vi "Main.vi"() -> ()   [LabVIEW 2020]
uses:
  controls/message cluster.ctl
  <vilib>/Platform/TimedLoop/XDataNode/timing_clust.ctl
  <vilib>/Platform/TimedLoop/XDataNode/nitl_modes.ctl
  <vilib>/Platform/TimedLoop/XDataNode/wakeup.ctl
  <instrlib>/Marlin Instrument Driver/Public/controls/move parameters.ctl
  <instrlib>/Marlin Instrument Driver/Public/controls/axes.ctl
  <instrlib>/Marlin Instrument Driver/Public/controls/heater.ctl
  <vilib>/Utility/config.llb/Read Key (String).vi
  <vilib>/Utility/config.llb/Read Key (Double).vi
  <vilib>/Utility/config.llb/Write Key (String).vi
  <vilib>/Utility/config.llb/Write Key (Double).vi
  <vilib>/platform/TimedLoop/XDataNode/XDataNode.xnode
  <instrlib>/Marlin Instrument Driver/Marlin Instrument Driver.lvlib
  <vilib>/Utility/config.llb/NI_LVConfig.lvlib
  <vilib>/Platform/TimedLoop/XDataNode/XDNodeRunTimeDep.lvlib
panel:
  in  "Tab Control":T1(tab)
  in  "Disable steppers":bool
  in  "Chamber temp":enum16{"0", "40", "50", "60", "70", "80"}(ring) caption="Enum"
  in  "Bed temp":enum16{"0", "50", "60", "80", "100", "120"}(ring) caption="Enum"
  in  "Nozzle temp":T2(ring) caption="Enum"
  in  "Speed":u32=1000 caption="mm/min"
  in  "Distance":enum16{"0.1", "1", "10", "100"}(ring)=enum."10" caption="mm"
  in  "Fan control":u8(slide) caption="%" scale=0.0..255.0
  in  "Extrude":bool
  in  "Retract":bool
  in  "Home all":bool caption="ALL"
  in  "Home Z":bool
  in  "Z-":bool
  in  "Z+":bool
  in  "Home XY":bool
  in  "XY-":bool
  in  "X-":bool
  in  "XY+":bool
  in  "X-Y+":bool
  in  "Y-":bool
  in  "X+Y-":bool
  in  "X+":bool
  in  "Y+":bool
  in  "Monitor data":bool caption="Monitoring slows down communication"
  in  "Update frequency":u32=1000 caption="ms"
  out "Temperature Chart":dbl[][](graph)
  out "Z min":bool
  out "Y min":bool
  out "X min":bool
  out "Gcode array":string[](array[string])
  in  "Stop Gcode":bool
  in  "Pause Gcode":bool
  in  "Test mode":bool
  out "XY Graph":cluster{"X":dbl, "Y":dbl}[](graph)
  in  "Start Gcode":bool
  in  "Gcode file":path caption="Path"
  out "Position sent":dbl caption="Numeric"
  in  "Test mode":bool
  in  "Start torture":bool
  in  "Axle":enum16{"X", "Y", "Z"}(ring) caption="Enum"
  in  "Speed":u32(slide)=3000 caption="%" scale=0.0..9000.0
  in  "Distance":dbl(slide)=100.0 caption="%" scale=0.0..235.0
  out "Initialized":bool
  in  "Initialize":bool
  in  "Delete":bool
  in  "Save":bool
  in  "Z":dbl caption="Numeric"
  in  "Y":dbl caption="Numeric"
  in  "X":dbl caption="Build volume"
  in  "COM port":refnum<visa-resource-name>
  in  "3D printer":string(combo) caption="Combo Box"
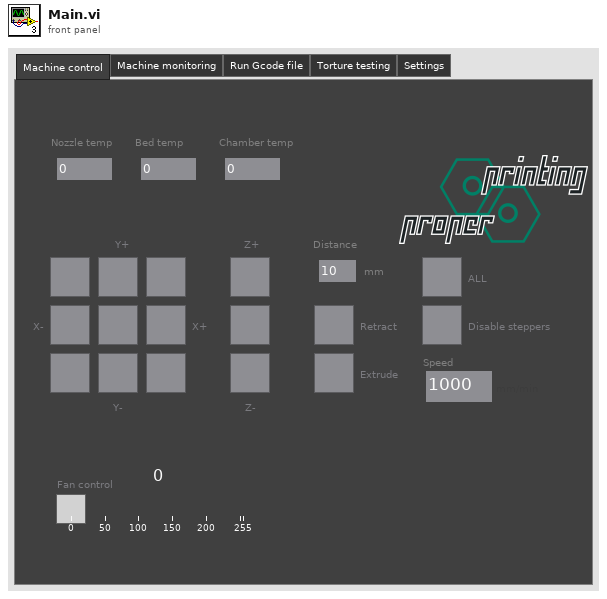
[diagram p1: front panel]
types:
  T1 = enum32{"Machine control", "Machine monitoring", "Run Gcode file", "Torture testing", "Settings"}
  T2 = enum16{"0", "100", "200", "230", "240", "260", "280", "290"}
  T3 = enum8{"Enabled", "Disabled", "Disabled and Grayed Out"}
  T4 = typedef "message cluster.ctl" = cluster{"message":string, "data":variant}
  T5 = typedef "XDNodeRunTimeDep.lvlib/timing_clust.ctl" = cluster{"Expected End [f-1]":u64, "Actual End [f-1]":u64, "Finished Late? [f-1]":bool, "Expected End [i-1]":u64, "Actual End [i-1]":u64, "Finished Late? [i-1]":bool, "Expected Start [i]":u64, "Actual Start [i]":u64, "Expected Start [f]":u64, "Actual Start [f]":u64, "Source Name":string, "Structure Name":string, "Period":i64, "Deadline":i64, "Offset":i64, "Start":i64, "Priority":i32, "Timeout":i32, "Mode":T6, "Wakeup Reason":T7, "Error":errorcluster, "Source Type":string, "Secondary Source Type":string, "Global End Time":u64, "Global Start Time":u64, "Frame Duration":u64, "Iteration Duration":u64, "Assigned CPU":i32, "I/O Scan Engine Mode":u32}
  T6 = typedef "XDNodeRunTimeDep.lvlib/nitl_modes.ctl" = enum32{"No Change", "Process missed periods, maintain original phase", "Discard missed periods, maintain original phase", "Process missed periods, ignore original phase", "Discard missed periods, ignore original phase"}
  T7 = typedef "XDNodeRunTimeDep.lvlib/wakeup.ctl" = enum32{"Normal", "Aborted", "Asynchronous wakeup", "Timing source error", "Timed loop error", "Timeout"}
  T8 = typedef "NI_LVConfig.lvlib/Config Data RefNum.ctl" = refnum<k1>
  T9 = typedef "Marlin Instrument Driver.lvlib/heater.ctl" = enum16{"Hot end", "Bed", "Chamber"}
  T10 = typedef "Marlin Instrument Driver.lvlib/move parameters.ctl" = cluster{"E":dbl, "F":dbl, "X":dbl, "Y":dbl, "Z":dbl}
  T11 = typedef "Marlin Instrument Driver.lvlib/axes.ctl" = cluster{"X":bool, "Y":bool, "Z":bool}
  T12 = typedef "Marlin Instrument Driver.lvlib/end stop status.ctl" = cluster{"x_min":bool, "y_min":bool, "z_min":bool}
  T13 = typedef "Marlin Instrument Driver.lvlib/temperatures.ctl" = cluster{"T":dbl, "T setpoint":dbl, "B":dbl, "B setpoint":dbl}
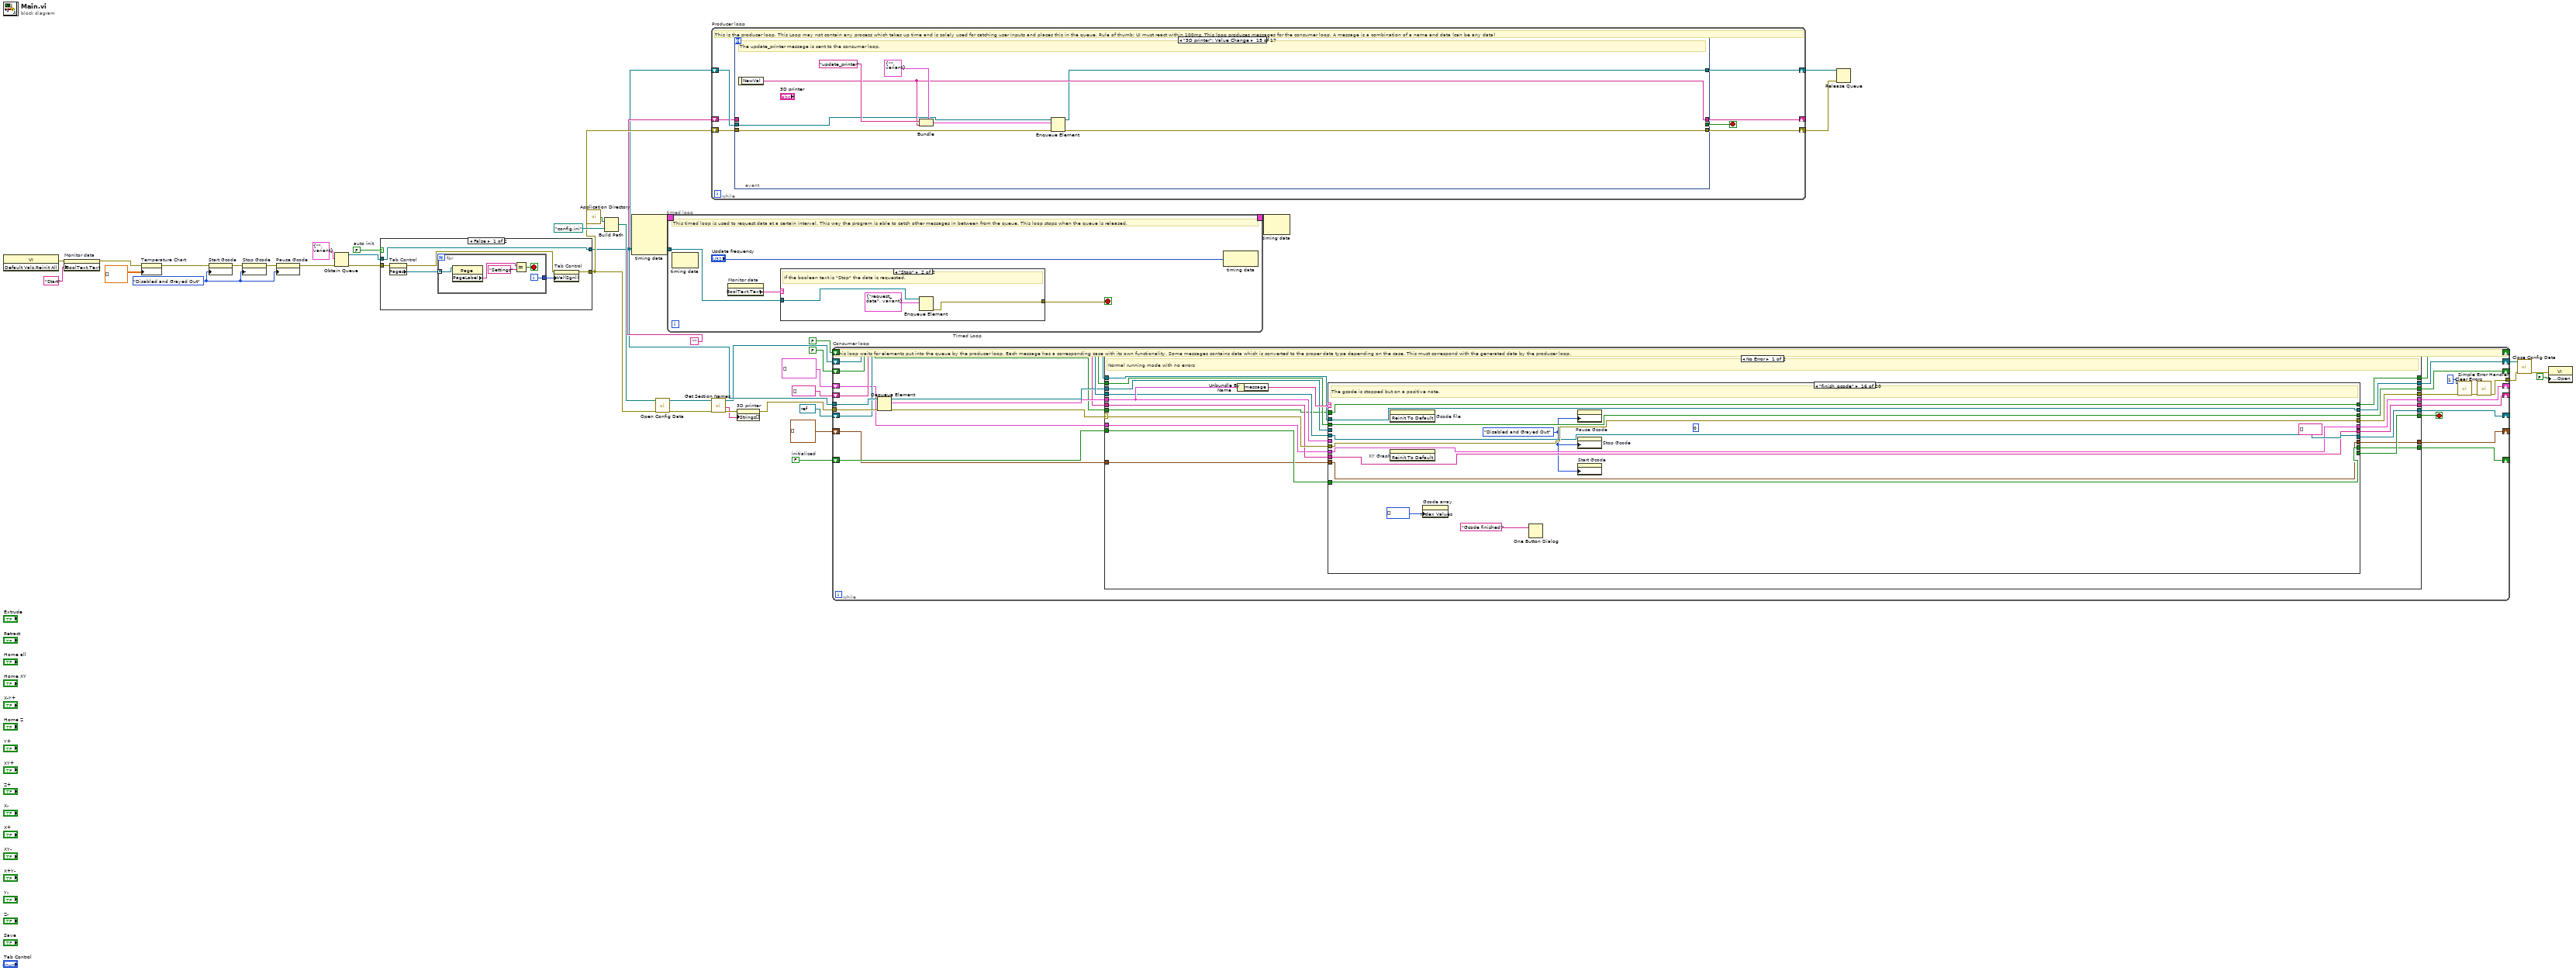
[diagram p0: block diagram]
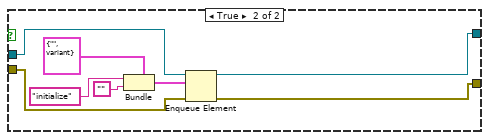
[diagram p2: hidden frame]
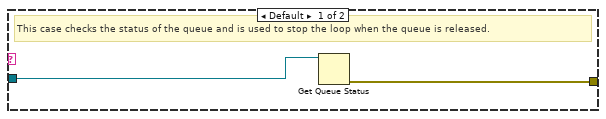
[diagram p3: hidden frame]
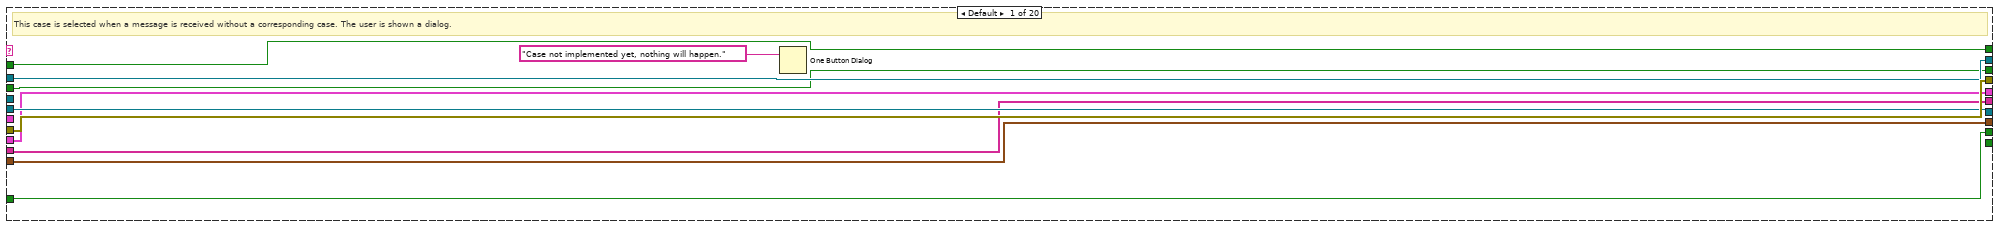
[diagram p4: hidden frame]
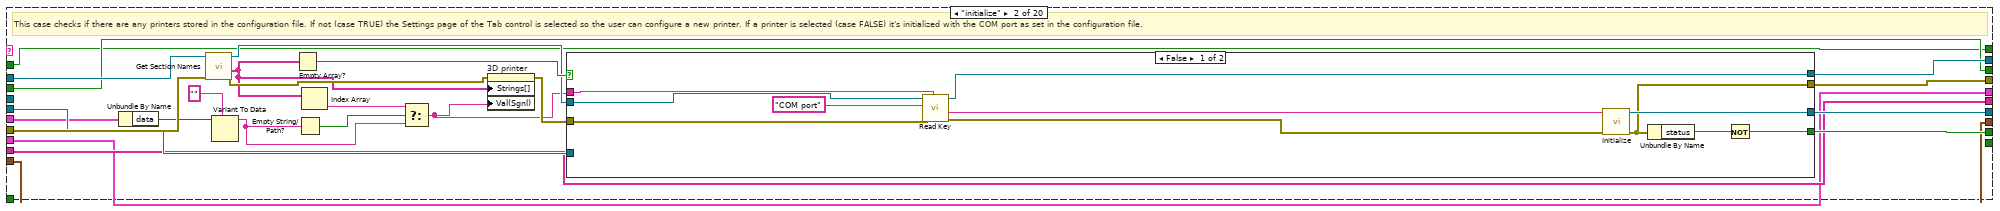
[diagram p5: hidden frame]
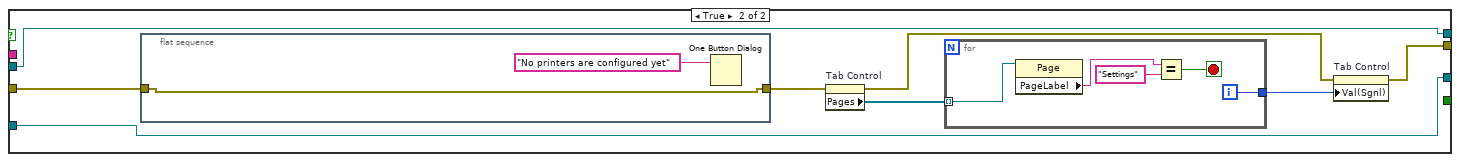
[diagram p6: hidden frame]
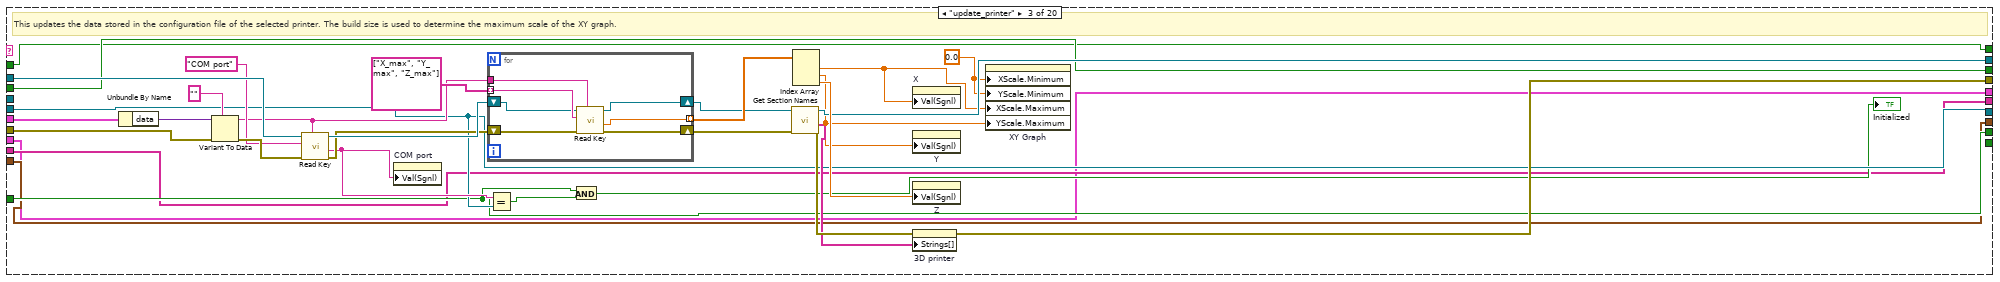
[diagram p7: hidden frame]
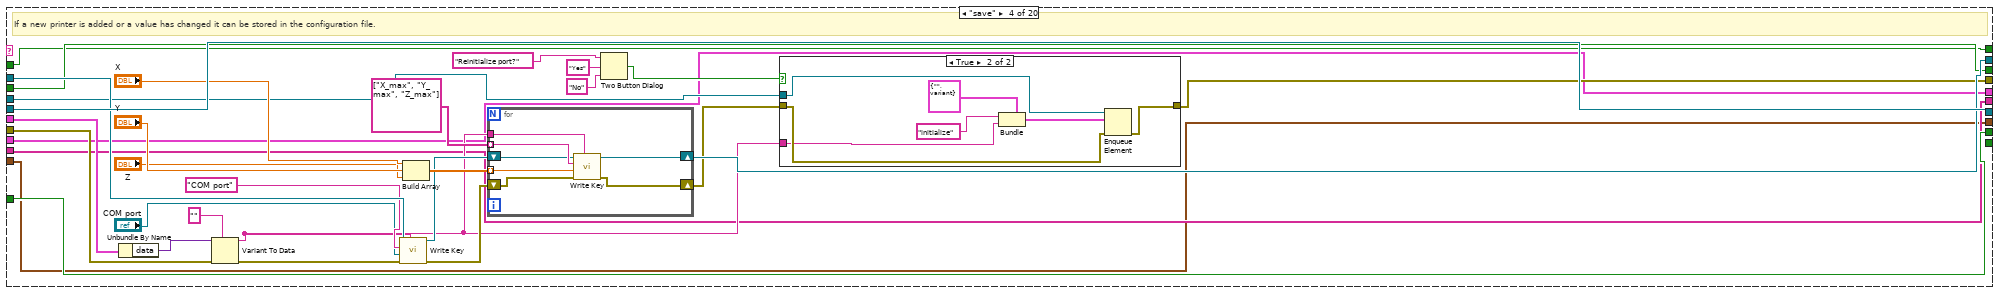
[diagram p8: hidden frame]
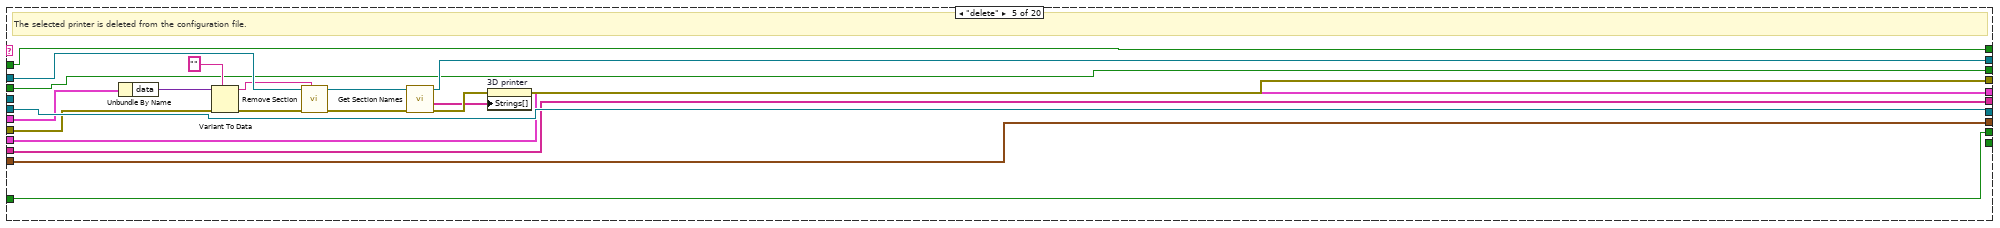
[diagram p10: hidden frame]
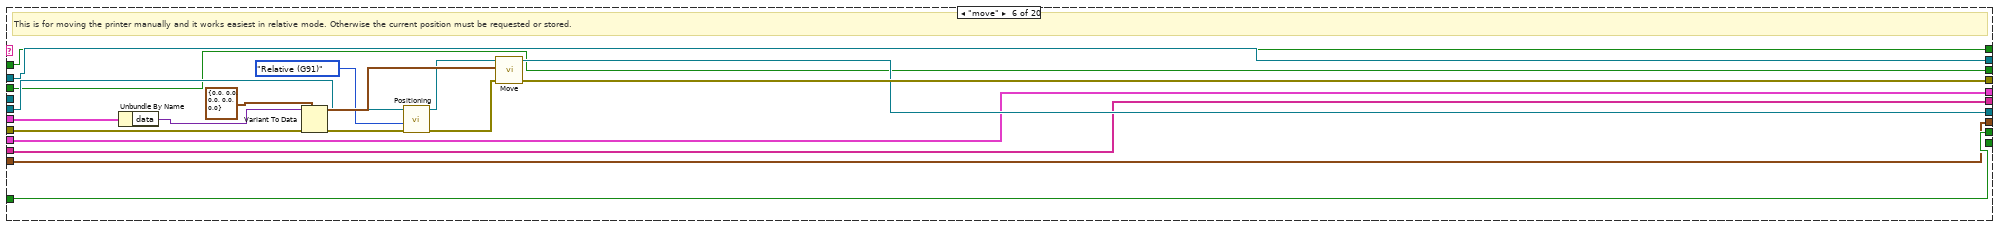
[diagram p11: hidden frame]
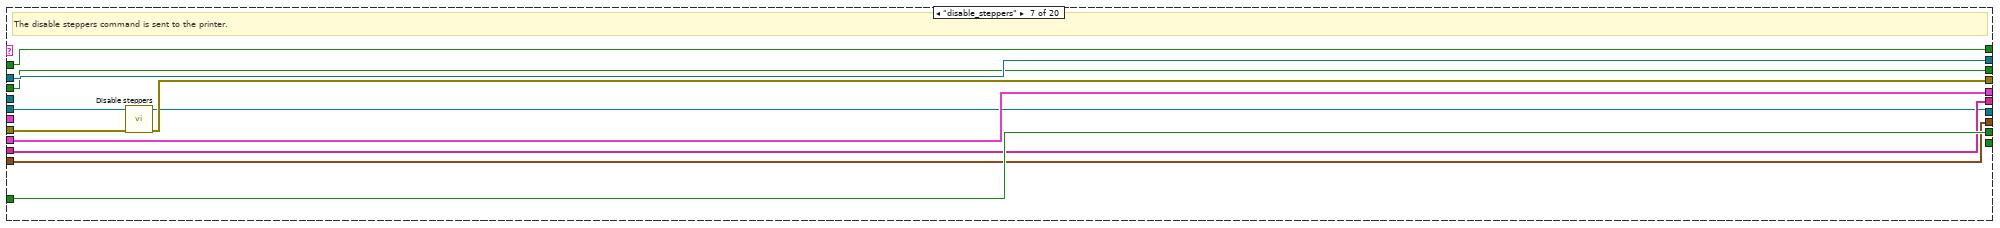
[diagram p12: hidden frame]
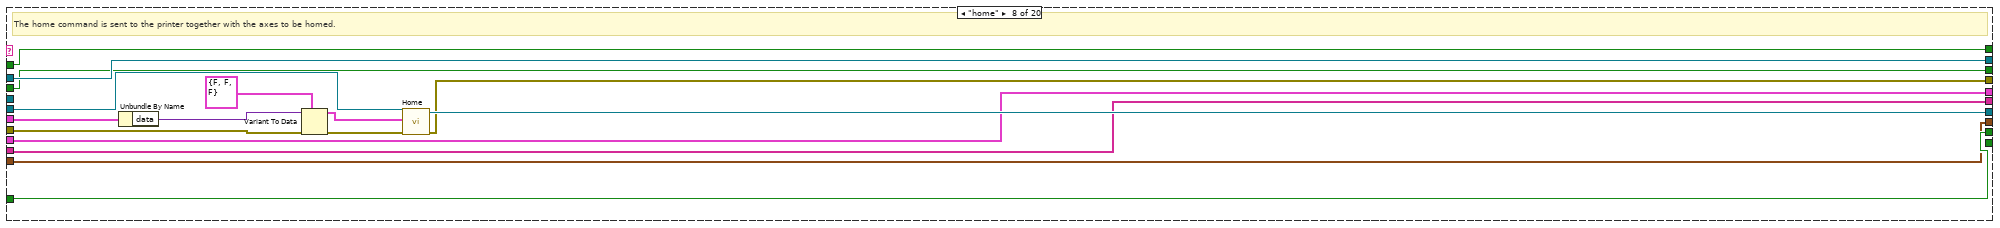
[diagram p13: hidden frame]
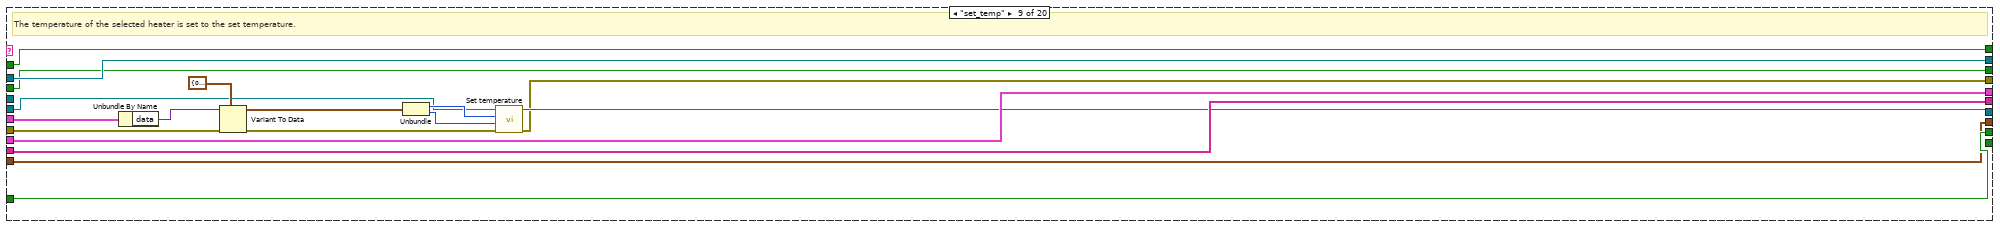
[diagram p14: hidden frame]
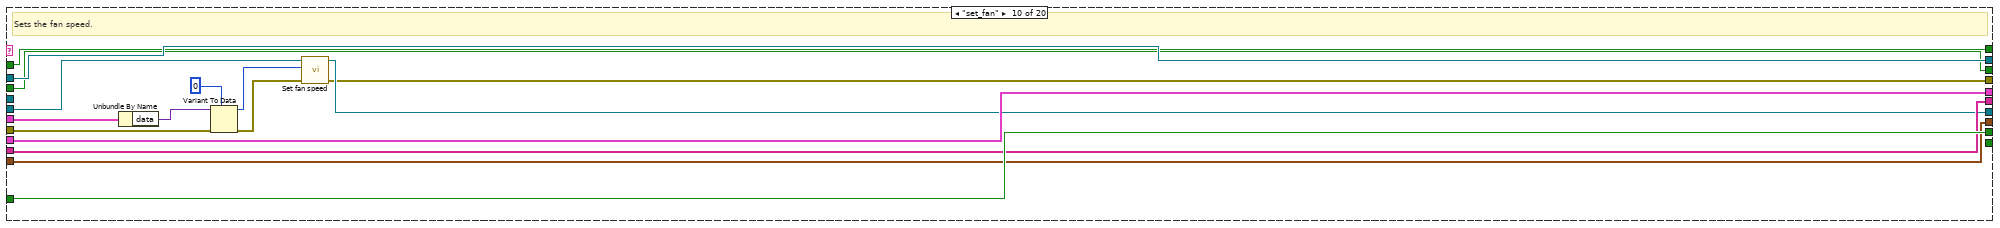
[diagram p15: hidden frame]
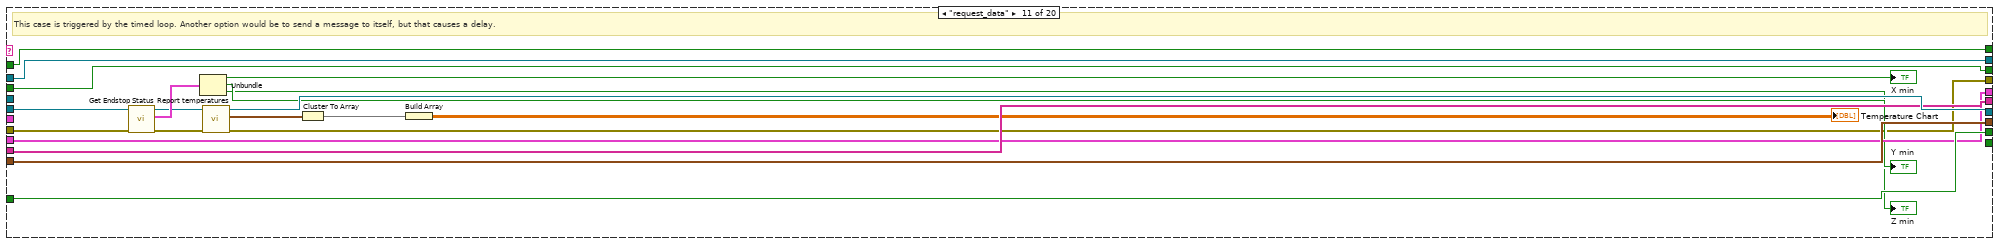
[diagram p16: hidden frame]
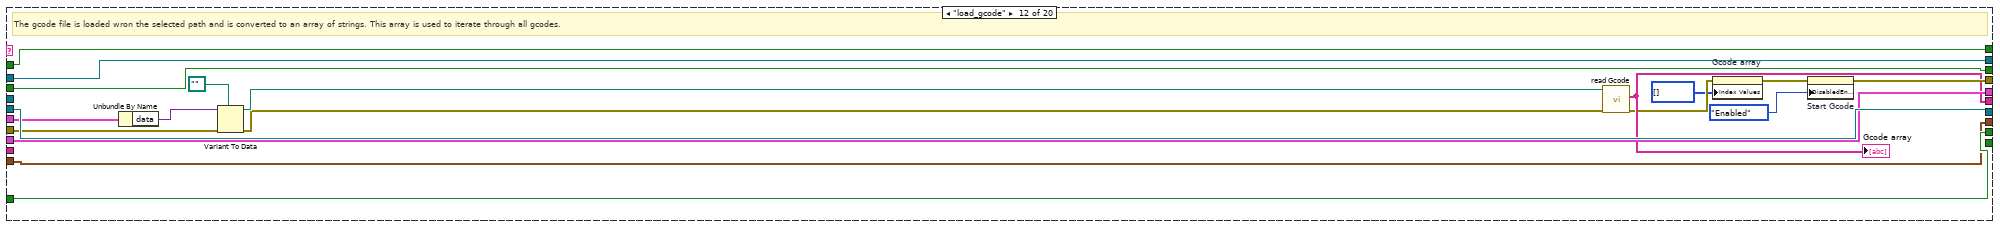
[diagram p17: hidden frame]
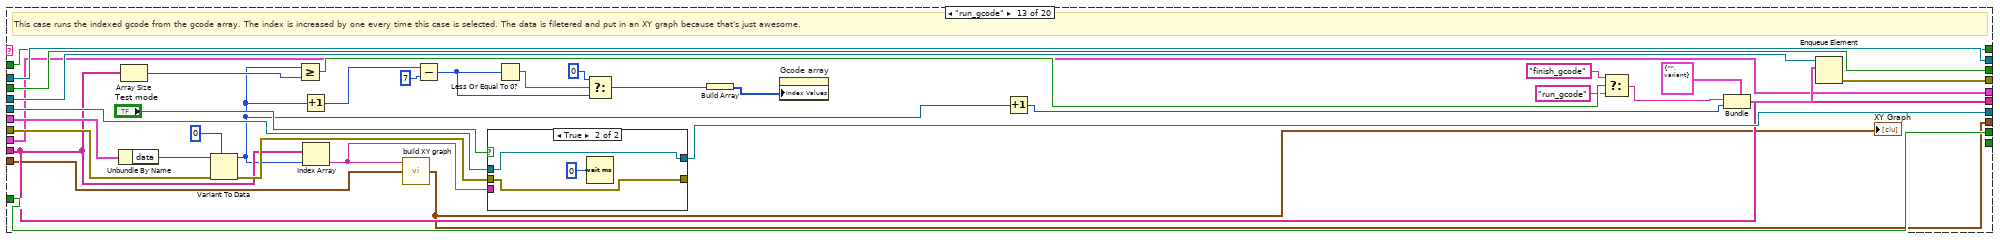
[diagram p18: hidden frame]
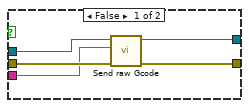
[diagram p19: hidden frame]
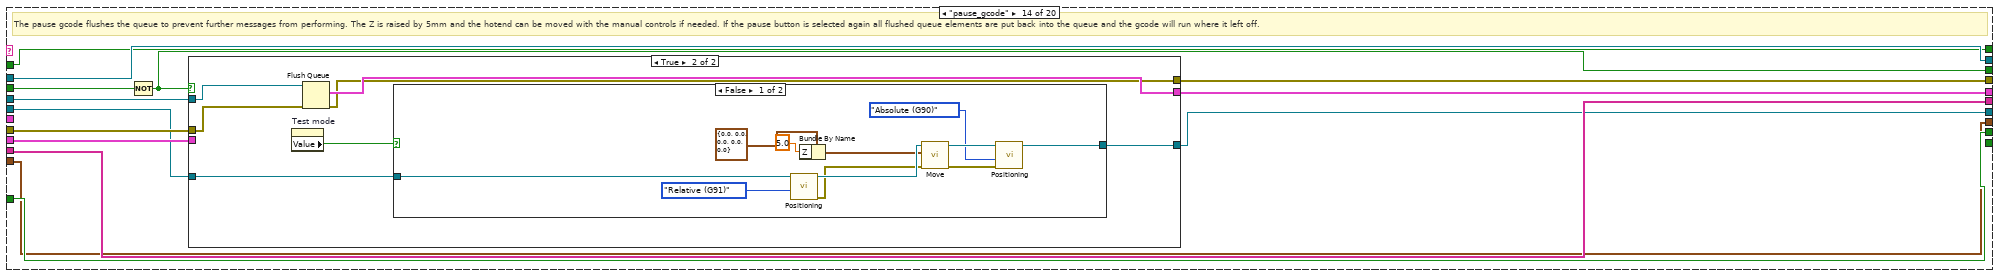
[diagram p20: hidden frame]
diagram:
  w15 = FALSE  # auto init
  w19 = T3."Disabled and Grayed Out" ("Disabled")
  w34 = FALSE  # initialized
  n1 = invoke class="VI" method="Default Vals.Reinit All"() -> (error out=w1:errorcluster)  [unwired: 3 in, 2 out]
  n2 = property on="Monitor data" class="Bool"(error in=w1, "BoolText.Text"="Start" ("Boolean Text.Text")) -> (error out=w11:errorcluster)  [unwired: 1 in, 1 out]
  n3 = property on="Temperature Chart" class="WFChart (strict)"(error in=w11, "History Data"=dbl[][] []) -> (error out=w14:errorcluster)  [unwired: 1 in, 1 out]
  n4 = property on="Start Gcode" class="Bool"(error in=w14, "DisabledEnum"=w19) -> (error out=w18:errorcluster)  [unwired: 1 in, 1 out]
  n5 = property on="Stop Gcode" class="Bool"(error in=w18, "DisabledEnum"=w19) -> (error out=w17:errorcluster)  [unwired: 1 in, 1 out]
  n6 = property on="Pause Gcode" class="Bool"(error in=w17, "DisabledEnum"=w19) -> (error out=w2:errorcluster)  [unwired: 1 in, 1 out]
  n7 = Obtain Queue(element data type=T4 {"message"="", "data"=variant}, error in (no error)=w2) -> (queue out=w37:refnum<queue>, error out=w36:errorcluster)  [unwired: 3 in, 1 out]
  n8 = case shown="False" w15 {
    tunnel: w37 -> [w46 w59]
    tunnel: w36 -> [w42 w58]
    tunnel: [w41 w57] -> w30
    tunnel: [w46 w52] -> w20
    frame False {
      n9 = property on="Tab Control" class="TabCtl (strict)"(error in=w42) -> (error out=w43:errorcluster, "Pages"=w44:refnum<vi>[])  [unwired: 1 in, 1 out]
      n10 = for {
        tunnel: w44 -> [w51] mode=indexing
        tunnel: [w47] -> w45
        i -> [w47]
        stop <- w48 stop-if-true
        n11 = property class="Page"(reference=w51) -> ("PageLabel"=w50:string)  [unwired: 1 in, 2 out]
        n12 = Equal?(x=w50, y="Settings") -> (x = y?=w48:bool)
      }
      n13 = property on="Tab Control" class="TabCtl (strict)"(error in=w43, "Val(Sgnl)"=w45) -> (error out=w41:errorcluster)  [unwired: 1 in, 1 out]
    }
    frame True {
      n14 = Bundle(cluster=T4 {"message"="", "data"=variant}, "message"="initialize", "data"="") -> (w53:T4)
      n15 = Enqueue Element(queue=w59, element=w53, error in (no error)=w58) -> (queue out=w52:refnum<queue>, error out=w57:errorcluster)  [unwired: 1 in, 1 out]
    }
  }
  n16 = call <vilib>:"Application Directory.vi"() -> ("Application Directory"=w33:path)
  n17 = Build Path(base path=w33, name or relative path=path "config.ini") -> (appended path=w31:path)
  n18 = node-c288() -> (w22:T5)  [unwired: 4 in]
  n19 = call <vilib>:"Open Config Data.vi"("error in (no error)"=w30, "configuration file path"=w31) -> ("error out"=w8:errorcluster, "refnum"=w7:T8)  [unwired: 7 in, 1 out]
  n20 = timed-loop "Timed Loop" {
    timing: w22 -> [_]
    timing-out: [_] -> w21
    tunnel: w20 -> [w62]
    stop <- w60 stop-if-true
    # "This timed loop is used to request data at a certain interval. This way the program is able to catch other messages in between from the queue. This loop stops when the queue is released."
    n21 = node-c288() -> ()  [unwired: 1 in, 1 out]
    n22 = property on="Monitor data" class="Bool"() -> ("BoolText.Text"=w61:string)  [unwired: 2 in, 2 out]
    n23 = case shown="\"Stop\"" w61 {
      tunnel: w62 -> [w64 w68]
      tunnel: [w65 w67] -> w60
      frame Default {
        # "This case checks the status of the queue and is used to stop the loop when the queue is released."
        n24 = Get Queue Status(queue=w64) -> (error out=w65:errorcluster)  [unwired: 2 in, 7 out]
      }
      frame "Stop" {
        # "If the boolean text is \"Stop\" the data is requested."
        n25 = Enqueue Element(queue=w68, element=T4 {"message"="request_data", "data"=variant}) -> (error out=w67:errorcluster)  [unwired: 2 in, 2 out]
      }
    }
    n26 = node-c288("Update frequency") -> ()  [unwired: 1 out]
  }
  n27 = while "Producer loop" {
    shift-right: [w76] -> w39
    shift-left: w30 -> [w77]
    shift-right: [w75] -> w38
    shift-left: w20 -> [w78]
    shift-right: [w74] -> _
    shift-left: "" -> [w73]
    stop <- w79 stop-if-true
    # "This is the producer loop. This Loop may not contain any process which takes up time and is solely used for catching user inputs and places this in the queue. Rule of thumb: UI must react within 100ms. This loop produces messages for the consumer loop. A message is a combination of a name and data (can be any data)"
    n28 = event shown="[14] \"3D printer\": Value Change" {
      selector: _ -> [_ _ _ _ _ _ _ _ _ _ _ _ _ _ _ _ _]
      dyn-events: _ -> [_ _ _ _ _ _ _ _ _ _ _ _ _ _ _ _ _]
      timeout: _ -> [_ _ _ _ _ _ _ _ _ _ _ _ _ _ _ _ _]
      tunnel: [_ _ _ _ _ _ _ _ _ _ _ _ _ _ _ _ TRUE] -> w79
      tunnel: w78 -> [w81 w87 w97 w125 w177 w187 w205 w219 w233 w242 w251 w270 w280 w296 w300 w308 w319]
      tunnel: w77 -> [w82 w86 w95 w120 w175 w185 w202 w217 w229 w239 w252 w268 w278 w294 w299 w307 w317]
      tunnel: [w82 w85 w94 w119 w174 w184 w201 w215 w224 w238 w246 w267 w277 w293 w298 w306 w316] -> w76
      tunnel: [w81 w84 w96 w121 w176 w186 w204 w218 w233 w240 w250 w269 w279 w295 w297 w305 w315] -> w75
      tunnel: [w80 w83 w107 w115 w179 w188 w211 w223 w235 w245 w254 w272 w281 w290 w301 w309 w314] -> w74
      tunnel: w73 -> [w80 w83 w107 w115 w179 w188 w211 w223 w235 w245 w254 w272 w281 w290 _ w309 w314]
      event Timeout {
        # "This event will never trigger (timeout = -1)"
        n29 = event-data() -> ()  [unwired: 1 in, 3 out]
      }
      event "Initialize": Value Change {
        # "The initialize message is sent to the consumer loop."
        n30 = event-data() -> ()  [unwired: 1 in, 6 out]
        n31 = Bundle(cluster=T4 {"message"="", "data"=variant}, "message"="initialize", "data"=w83) -> (w88:T4)
        n32 = Enqueue Element(queue=w87, element=w88, error in (no error)=w86) -> (queue out=w84:refnum<queue>, error out=w85:errorcluster)  [unwired: 1 in, 1 out]
      }
      event "Nozzle temp", "Bed temp", "Chamber temp": Value Change {
        # "This event looks at the lable of which input has changed which corresponds with a case. The data is sent together with the set_temp message to the consumer loop."
        n33 = event-data() -> ("CtlRef"=w106:refnum<vi>)  [unwired: 1 in]
        n34 = property class="Enum"(reference=w106) -> ("Label.Text"=w105:string, "Strings []"=w104:string[])  [unwired: 1 in, 2 out]
        n35 = case shown="\"Chamber temp\"" w105 {
          tunnel: ["Bed temp" "Chamber temp" "Nozzle temp"] -> w103
          tunnel: [heater."Bed" ("Heater") heater."Chamber" ("Heater") heater."Hot end" ("Heater")] -> w91
          frame "Bed temp" {
          }
          frame "Chamber temp" {
          }
          frame "Nozzle temp", Default {
          }
        }
        n36 = Index Array(array=w104, index=w103) -> (element=w102:string)
        n37 = Decimal String To Number(string=w102) -> (number=w101:i32)  [unwired: 2 in, 1 out]
        n38 = Bundle(cluster=cluster{"setpoint":i32, "Heater":T9} {"setpoint"=0, "Heater"=enum."Hot end"} ("output cluster"), "setpoint"=w101, "Heater"=w91) -> (w93:cluster{"setpoint":i32, "Heater":T9})
        n39 = Bundle(cluster=T4 {"message"="", "data"=variant}, "message"="set_temp", "data"=w93) -> (w98:T4)
        n40 = Enqueue Element(queue=w97, element=w98, error in (no error)=w95) -> (queue out=w96:refnum<queue>, error out=w94:errorcluster)  [unwired: 1 in, 1 out]
      }
      event "Y+", "X+", "X+Y-", "Y-", "X-Y+", "XY+", "X-", "XY-", "Z+", "Z-", "Extrude", "Retract": Value Change {
        # "Depending on which button is pressed the matching case is selected. This sends the value with the move message. This only works with relative positioning because the unused values are 0."
        n41 = event-data() -> ("CtlRef"=w130:refnum<vi>)  [unwired: 1 in]
        n42 = property class="Bool"(reference=w130) -> ("Label.Text"=w129:string)  [unwired: 1 in, 2 out]
        n43 = property on="Distance" class="Enum (strict)"() -> ("Strings []"=w128:string[])  [unwired: 2 in, 2 out]
        n44 = Index Array(array=w128, index="Distance") -> (element=w127:string)
        n45 = Fract/Exp String To Number(string=w127) -> (number=w126:dbl)  [unwired: 3 in, 1 out]
        n46 = case shown="\"X+Y-\"" w129 {
          tunnel: w126 -> [_ w132 w135 w138 w141 w145 w149 w152 w156 w159 w163 w167 w171]
          tunnel: [_ w131 w134 w137 w142 w146 w150 w153 w157 w161 w165 w168 w172] -> w118
          frame Default {
          }
          frame "X+" {
            n47 = Bundle By Name(cluster=T10 {"E"=0.0, "F"=0.0, "X"=0.0, "Y"=0.0, "Z"=0.0} ("Distances"), "X"=w132) -> (w131:T10)
          }
          frame "Y+" {
            n48 = Bundle By Name(cluster=T10 {"E"=0.0, "F"=0.0, "X"=0.0, "Y"=0.0, "Z"=0.0} ("Distances"), "Y"=w135) -> (w134:T10)
          }
          frame "Z+" {
            n49 = Bundle By Name(cluster=T10 {"E"=0.0, "F"=0.0, "X"=0.0, "Y"=0.0, "Z"=0.0} ("Distances"), "Z"=w138) -> (w137:T10)
          }
          frame "X-" {
            n50 = Negate(x=w141) -> (-x=w140:dbl)
            n51 = Bundle By Name(cluster=T10 {"E"=0.0, "F"=0.0, "X"=0.0, "Y"=0.0, "Z"=0.0} ("Distances"), "X"=w140) -> (w142:T10)
          }
          frame "Y-" {
            n52 = Negate(x=w145) -> (-x=w144:dbl)
            n53 = Bundle By Name(cluster=T10 {"E"=0.0, "F"=0.0, "X"=0.0, "Y"=0.0, "Z"=0.0} ("Distances"), "Y"=w144) -> (w146:T10)
          }
          frame "Z-" {
            n54 = Negate(x=w149) -> (-x=w148:dbl)
            n55 = Bundle By Name(cluster=T10 {"E"=0.0, "F"=0.0, "X"=0.0, "Y"=0.0, "Z"=0.0} ("Distances"), "Z"=w148) -> (w150:T10)
          }
          frame "XY+" {
            n56 = Bundle By Name(cluster=T10 {"E"=0.0, "F"=0.0, "X"=0.0, "Y"=0.0, "Z"=0.0} ("Distances"), "X"=w152, "Y"=w152) -> (w153:T10)
          }
          frame "XY-" {
            n57 = Negate(x=w156) -> (-x=w155:dbl)
            n58 = Bundle By Name(cluster=T10 {"E"=0.0, "F"=0.0, "X"=0.0, "Y"=0.0, "Z"=0.0} ("Distances"), "X"=w155, "Y"=w155) -> (w157:T10)
          }
          frame "X+Y-" {
            n59 = Negate(x=w159) -> (-x=w160:dbl)
            n60 = Bundle By Name(cluster=T10 {"E"=0.0, "F"=0.0, "X"=0.0, "Y"=0.0, "Z"=0.0} ("Distances"), "X"=w159, "Y"=w160) -> (w161:T10)
          }
          frame "X-Y+" {
            n61 = Negate(x=w163) -> (-x=w164:dbl)
            n62 = Bundle By Name(cluster=T10 {"E"=0.0, "F"=0.0, "X"=0.0, "Y"=0.0, "Z"=0.0} ("Distances"), "X"=w164, "Y"=w163) -> (w165:T10)
          }
          frame "Extrude" {
            n63 = Bundle By Name(cluster=T10 {"E"=0.0, "F"=0.0, "X"=0.0, "Y"=0.0, "Z"=0.0} ("Distances"), "E"=w167) -> (w168:T10)
          }
          frame "Retract" {
            n64 = Negate(x=w171) -> (-x=w170:dbl)
            n65 = Bundle By Name(cluster=T10 {"E"=0.0, "F"=0.0, "X"=0.0, "Y"=0.0, "Z"=0.0} ("Distances"), "E"=w170) -> (w172:T10)
          }
        }
        n66 = Bundle By Name(cluster=w118, "F"="Speed") -> (w117:T10)
        n67 = Bundle(cluster=T4 {"message"="", "data"=variant}, "message"="move", "data"=w117) -> (w124:T4)
        n68 = Enqueue Element(queue=w125, element=w124, error in (no error)=w120) -> (queue out=w121:refnum<queue>, error out=w119:errorcluster)  [unwired: 1 in, 1 out]
      }
      event "Disable steppers": Value Change {
        # "The disable_steppers message is sent to the consumer loop."
        n69 = event-data() -> ()  [unwired: 1 in, 6 out]
        n70 = Enqueue Element(queue=w177, element=T4 {"message"="disable_steppers", "data"=variant}, error in (no error)=w175) -> (queue out=w176:refnum<queue>, error out=w174:errorcluster)  [unwired: 1 in, 1 out]
      }
      event "Start torture": Value Change {
        # "Depending on the boolean text the start_torture or stop_torture  message is sent to the consumer loop. The boolean text is changed from start to stop and vice versa when pressed."
        n71 = event-data() -> ("CtlRef"=w183:refnum<vi>)  [unwired: 1 in, 5 out]
        n72 = property class="Bool"(reference=w183) -> (reference out=w181:refnum<vi>, "BoolText.Text"=w182:string)  [unwired: 1 in, 1 out]
        n73 = case shown="\"Start\"" w182 {
          tunnel: w187 -> [w193 w199]
          tunnel: [w192 w198] -> w186
          tunnel: w185 -> [w191 w197]
          tunnel: [w190 w196] -> w184
          tunnel: ["Stop" "Start"] -> w180
          frame "Start" {
            n74 = Enqueue Element(queue=w193, element=T4 {"message"="start_torture", "data"=variant}, error in (no error)=w191) -> (queue out=w192:refnum<queue>, error out=w190:errorcluster)  [unwired: 1 in, 1 out]
          }
          frame "Stop", Default {
            n75 = Enqueue Element At Opposite End(queue=w199, element=T4 {"message"="stop_torture", "data"=variant}, error in (no error)=w197) -> (queue out=w198:refnum<queue>, error out=w196:errorcluster)  [unwired: 1 in, 1 out]
          }
        }
        n76 = property class="Bool"(reference=w181, "BoolText.Text"=w180) -> ()  [unwired: 1 in, 2 out]
      }
      event "Home XY", "Home Z", "Home all": Value Change {
        # "The home message is sent to the consumer loop together with the data which tells which axes to home."
        n77 = event-data() -> ("CtlRef"=w210:refnum<vi>)  [unwired: 1 in]
        n78 = property class="Bool"(reference=w210) -> ("Label.Text"=w209:string)  [unwired: 1 in, 2 out]
        n79 = case shown="\"Home Z\"" w209 {
          tunnel: [T11 {"X"=TRUE, "Y"=TRUE, "Z"=TRUE} ("Axes") T11 {"X"=TRUE, "Y"=TRUE, "Z"=FALSE} ("Axes") T11 {"X"=FALSE, "Y"=FALSE, "Z"=TRUE} ("Axes")] -> w203
          frame "Home all", Default {
          }
          frame "Home XY" {
          }
          frame "Home Z" {
          }
        }
        n80 = Bundle(cluster=T4 {"message"="", "data"=variant}, "message"="home", "data"=w203) -> (w206:T4)
        n81 = Enqueue Element(queue=w205, element=w206, error in (no error)=w202) -> (queue out=w204:refnum<queue>, error out=w201:errorcluster)  [unwired: 1 in, 1 out]
      }
      event "Fan control": Value Change {
        # "The set_fan message is sent to the consumer loop. The NewVal is used and the event is triggered immediately when the Fan control slider is moved. This slows down communication and should therefore not be performed when a Gcode is running."
        n82 = event-data() -> ("NewVal"=w216:u8)  [unwired: 1 in]
        n83 = Bundle(cluster=T4 {"message"="", "data"=variant}, "message"="set_fan", "data"=w216) -> (w220:T4)
        n84 = Enqueue Element(queue=w219, element=w220, error in (no error)=w217) -> (queue out=w218:refnum<queue>, error out=w215:errorcluster)  [unwired: 1 in, 1 out]
      }
      event "Monitor data": Value Change {
        w227 = "Start" ("y")
        # "This event changes the boolean text of the Monitor data button from Start to Stop and vice versa. This is used to enable or disable the timed loop data request."
        n85 = event-data() -> ("CtlRef"=w234:refnum<vi>)  [unwired: 1 in, 2 out]
        n86 = property class="Bool"(reference=w234, error in=w229) -> (reference out=w231:refnum<vi>, error out=w230:errorcluster, "BoolText.Text"=w232:string)
        n87 = Equal?(x=w232, y=w227) -> (x = y?=w228:bool)
        n88 = Select(t="Stop", s=w228, f=w227) -> (s? t:f=w225:string)
        n89 = property class="Bool"(reference=w231, error in=w230, "BoolText.Text"=w225) -> (error out=w224:errorcluster)  [unwired: 1 out]
      }
      event "Gcode file": Value Change {
        # "The load_gcode message is sent to the consumer loop together with the selected path."
        n90 = event-data() -> ("NewVal"=w237:path)  [unwired: 1 in]
        n91 = Strip Path(path=w237) -> (name=w236:string)  [unwired: 1 out]
        n92 = property on="Gcode file" class="Path"("Text.Text"=w236) -> ()  [unwired: 2 in, 2 out]
        n93 = Bundle(cluster=T4 {"message"="", "data"=variant} ("element"), "message"="load_gcode", "data"=w237) -> (w241:T4)
        n94 = Enqueue Element(queue=w242, element=w241, error in (no error)=w239) -> (queue out=w240:refnum<queue>, error out=w238:errorcluster)  [unwired: 1 in, 1 out]
      }
      event "Start Gcode": Value Change {
        # "The run_gcode message is sent to the consumer loop after the user confirms the message. The current index of the Gcode array (first array element is 0) is sent as data."
        n95 = event-data() -> ()  [unwired: 1 in, 4 out]
        n96 = Two Button Dialog(message="Run selected program?", 1:"No" ("F button name (\"Cancel\")"), 2:"Yes" ("T button name (\"OK\")")) -> (T button?=w249:bool)
        n97 = case shown="True" w249 {
          tunnel: w252 -> [w255 w263]
          tunnel: w251 -> [w256 w262]
          tunnel: [w256 w261] -> w250
          tunnel: [w255 w259] -> w246
          frame False {
          }
          frame True {
            w257 = T3."Enabled" ("Disabled")
            n98 = property on="Stop Gcode" class="Bool"("DisabledEnum"=w257) -> ()  [unwired: 2 in, 2 out]
            n99 = property on="Pause Gcode" class="Bool"("DisabledEnum"=w257) -> ()  [unwired: 2 in, 2 out]
            n100 = Bundle(cluster=T4 {"message"="", "data"=variant} ("element"), "message"="run_gcode", "data"=0) -> (w264:T4)
            n101 = property on="Start Gcode" class="Bool"("DisabledEnum"=T3."Disabled and Grayed Out" ("Disabled")) -> ()  [unwired: 2 in, 2 out]
            n102 = Enqueue Element(queue=w262, element=w264, error in (no error)=w263) -> (queue out=w261:refnum<queue>, error out=w259:errorcluster)  [unwired: 1 in, 1 out]
          }
        }
      }
      event "Pause Gcode": Value Change {
        # "The pause_gcode message is sent to the consumer loop."
        n103 = event-data() -> ()  [unwired: 1 in, 1 out]
        n104 = Enqueue Element(queue=w270, element=T4 {"message"="pause_gcode", "data"=variant}, error in (no error)=w268) -> (queue out=w269:refnum<queue>, error out=w267:errorcluster)  [unwired: 1 in, 1 out]
      }
      event "Stop Gcode": Value Change {
        # "The stop_gcode message is sent to the consumer loop after the user confirms the message."
        n105 = event-data() -> ()  [unwired: 1 in, 1 out]
        n106 = Two Button Dialog(message="Stop current running program?", 1:"No" ("F button name (\"Cancel\")"), 2:"Yes" ("T button name (\"OK\")")) -> (T button?=w273:bool)
        n107 = case shown="True" w273 {
          tunnel: w280 -> [w283 w287]
          tunnel: [w283 w286] -> w279
          tunnel: w278 -> [w282 w285]
          tunnel: [w282 w284] -> w277
          frame False {
          }
          frame True {
            n108 = Enqueue Element At Opposite End(queue=w287, element=T4 {"message"="stop_gcode", "data"=variant}, error in (no error)=w285) -> (queue out=w286:refnum<queue>, error out=w284:errorcluster)  [unwired: 1 in, 1 out]
          }
        }
      }
      event "Save": Value Change {
        # "The save message is sent to the consumer loop."
        n109 = event-data() -> ()  [unwired: 1 in, 6 out]
        n110 = Bundle(cluster=T4 {"message"="", "data"=variant}, "message"="save", "data"=w290) -> (w289:T4)
        n111 = Enqueue Element(queue=w296, element=w289, error in (no error)=w294) -> (queue out=w295:refnum<queue>, error out=w293:errorcluster)  [unwired: 1 in, 1 out]
      }
      event "3D printer": Value Change {
        # "The update_printer message is sent to the consumer loop."
        n112 = event-data() -> ("NewVal"=w301:string)  [unwired: 1 in]
        n113 = Bundle(cluster=T4 {"message"="", "data"=variant}, "message"="update_printer", "data"=w301) -> (w302:T4)
        n114 = Enqueue Element(queue=w300, element=w302, error in (no error)=w299) -> (queue out=w297:refnum<queue>, error out=w298:errorcluster)  [unwired: 1 in, 1 out]
      }
      event "Delete": Value Change {
        # "The delete message is sent to the consumer loop."
        n115 = event-data() -> ()  [unwired: 1 in, 1 out]
        n116 = Bundle(cluster=T4 {"message"="", "data"=variant}, "message"="delete", "data"=w309) -> (w310:T4)
        n117 = Enqueue Element(queue=w308, element=w310, error in (no error)=w307) -> (queue out=w305:refnum<queue>, error out=w306:errorcluster)  [unwired: 1 in, 1 out]
      }
      event Panel Close? {
        # "The close message is sent to the consumer loop when the front panel is closed by the user. The message is discarded so the program can close the port first. The program quits after all loops are stopped."
        n118 = event-data() -> ()  [unwired: 1 in, 4 out]
        n119 = Enqueue Element(queue=w319, element=T4 {"message"="close", "data"=variant}, error in (no error)=w317) -> (queue out=w315:refnum<queue>, error out=w316:errorcluster)  [unwired: 1 in, 1 out]
        n120 = event-data("Discard?"=TRUE) -> ()  [unwired: 1 in, 1 out]
      }
    }
  }
  n121 = call <vilib>:"Get Section Names.vi"("error in (no error)"=w8, "refnum"=w7) -> ("error out"=w4:errorcluster, "section names"=w3:string[], "refnum out"=w6:T8)  [unwired: 7 in]
  n122 = property on="3D printer" class="CmbBox"(error in=w4, "Strings[]"=w3) -> (error out=w5:errorcluster)  [unwired: 1 in, 1 out]
  n123 = while "Consumer loop" {
    tunnel: w20 -> [w346]
    shift-right: [w341] -> _
    shift-left: refnum<visa-resource-name> refnum ("VISA resource name out") -> [w339]
    shift-right: [w340] -> w29
    shift-left: w6 -> [w338]
    shift-right: [w337] -> _
    shift-left: w34 -> [w336]
    shift-right: [w334] -> _
    shift-left: string[] [] ("Gcode Array") -> [w333]
    shift-right: [w331] -> _
    shift-left: cluster{"X":dbl, "Y":dbl}[] [] ("XY Graph 2") -> [w332]
    shift-right: [w326] -> _
    shift-left: FALSE -> [w327]
    shift-right: [w325] -> _
    shift-left: T4[] [] ("remaining elements") -> [w324]
    tunnel: w5 -> [w342]
    tunnel: [w323] -> w27
    shift-right: [w321] -> _
    shift-left: FALSE -> [w322]
    stop <- w344 stop-if-true
    # "This loop waits for elements put into the queue by the producer loop. Each message has a corresponding case with its own functionality. Some messages contains data which is converted to the proper data type depending on the case. This must correspond with the generated data by the producer loop."
    n124 = Dequeue Element(queue=w346, error in (no error)=w342) -> (queue out=w335:refnum<queue>, element=w345:T4, error out=w343:errorcluster)  [unwired: 1 in, 1 out]
    n125 = case shown="No Error" w343 {
      selector: w343 -> [w365 _]
      tunnel: w345 -> [w367 _]
      tunnel: [w366 FALSE] -> w344
      tunnel: [w364 w899] -> w341
      tunnel: [w363 w898] -> w340
      tunnel: w339 -> [w362 w899]
      tunnel: w338 -> [w361 w898]
      tunnel: [w360 _] -> w337
      tunnel: w336 -> [w359 _]
      tunnel: w335 -> [w358 w890]
      tunnel: [w357 w889] -> w330
      tunnel: [w356 w896] -> w334
      tunnel: w333 -> [w355 w896]
      tunnel: w332 -> [w354 w895]
      tunnel: [w353 w895] -> w331
      tunnel: w327 -> [w352 w894]
      tunnel: [w351 w894] -> w326
      tunnel: [w350 w893] -> w325
      tunnel: w324 -> [w349 w893]
      tunnel: w322 -> [w348 w892]
      tunnel: [w347 w892] -> w321
      frame No Error {
        # "Normal running mode with no errors"
        n126 = Unbundle By Name(w367) -> ("message"=w368:string)
        n127 = case shown="\"finish_gcode\"" w368 {
          tunnel: w367 -> [_ w391 w458 w482 w525 w552 _ w574 w591 w607 _ w649 w684 _ _ _ _ _ _ _]
          tunnel: [_ _ _ _ _ _ _ _ _ _ _ _ _ _ _ _ _ _ _ TRUE] -> w366
          tunnel: [w378 w399 w442 w483 w519 w548 w555 w569 w583 w603 w614 w639 w676 w699 w742 w760 w764 w823 w867 w878] -> w357
          tunnel: w365 -> [w378 w396 w457 w479 w528 w547 w556 w575 w582 w602 w616 w644 w683 w700 w743 w760 w769 w828 w868 w879]
          tunnel: [w376 w400 w440 w498 w533 w546 w554 w570 w584 w604 w630 w652 w679 w696 w748 w759 w762 w826 w877 w880] -> w364
          tunnel: [w377 w398 w444 w486 w520 w545 w563 w579 w597 w613 w633 w651 w687 w709 w747 w758 w776 w836 w876 w887] -> w363
          tunnel: w362 -> [w376 w394 w440 w498 w533 w541 w557 w577 w585 w605 w631 w652 w681 w697 w748 w759 w770 w827 w877 w880]
          tunnel: w361 -> [w377 w395 w455 w496 w531 w545 w563 w579 w597 w613 w633 w651 w687 w709 w747 w758 w776 w836 w876 w887]
          tunnel: [w375 w397 w439 w497 w532 w544 w562 w578 w596 w612 w632 w650 w686 w708 w746 w757 w775 w835 w875 w886] -> w360
          tunnel: w359 -> [w375 _ w439 w497 w532 w544 w562 w578 w596 w612 w632 w650 w686 w708 w746 w757 w775 w835 w875 w886]
          tunnel: w358 -> [_ _ _ w485 _ _ _ _ _ _ _ _ w675 w704 w744 _ w766 w822 w869 _]
          tunnel: [w374 w383 w436 w472 w518 w538 w561 w568 w595 w611 w629 w637 w674 w707 _ w756 w774 w834 w874 w885] -> w356
          tunnel: w355 -> [w374 w383 w436 w472 w518 w538 w561 w568 w595 w611 w629 _ w674 w707 _ w756 w774 w834 w874 w885]
          tunnel: w354 -> [w373 w382 w435 w471 w517 w537 w560 w567 w594 w610 w628 w643 w667 w706 w745 w754 w773 w833 w873 w884]
          tunnel: [w373 w382 w435 w471 w517 w537 w560 w567 w594 w610 w628 w643 w665 w706 w745 w754 w773 w833 w873 w884] -> w353
          tunnel: w352 -> [w372 w381 w431 w470 w516 w536 w559 w566 w593 w609 w627 w642 w657 w705 w741 w753 w772 w832 w872 w883]
          tunnel: [w372 w381 w431 w470 w516 w536 w559 w566 w593 w609 w627 w642 w657 w703 w741 w753 w772 w832 w872 w883] -> w351
          tunnel: [w371 w380 w430 w469 w515 w535 w558 w565 w592 w608 w626 w641 w656 w702 _ w752 w771 w831 w871 w882] -> w350
          tunnel: w349 -> [w371 w380 w430 w469 w515 w535 w558 w565 w592 w608 w626 w641 w656 w701 _ w752 w771 w831 w871 w882]
          tunnel: w348 -> [w370 w379 w429 w468 w514 w534 w553 w564 w580 w598 w615 w638 w655 w698 w739 w750 _ w816 w870 w881]
          tunnel: [w370 w379 w429 w468 w514 w534 w553 w564 w580 w598 w615 w638 w655 w698 w739 w750 FALSE w815 w870 w881] -> w347
          frame Default {
            # "This case is selected when a message is received without a corresponding case. The user is shown a dialog."
            n128 = One Button Dialog(message="Case not implemented yet, nothing will happen.") -> ()  [unwired: 1 in, 1 out]
          }
          frame "initialize" {
            # "This case checks if there are any printers stored in the configuration file. If not (case TRUE) the Settings page of the Tab control is selected so the user can configure a new printer. If a printer is selected (case FALSE) it's initialized with the COM port as set in the configuration file."
            n129 = Unbundle By Name(w391) -> ("data"=w393:variant)
            n130 = call <vilib>:"Get Section Names.vi"("error in (no error)"=w396, "refnum"=w395) -> ("error out"=w388:errorcluster, "section names"=w386:string[], "refnum out"=w401:T8)  [unwired: 7 in]
            n131 = Variant To Data(type="", Variant=w393) -> (data=w389:string)  [unwired: 1 in, 1 out]
            n132 = Empty Array?(array=w386) -> (empty?=w402:bool)
            n133 = Empty String/Path?(string/path=w389) -> (empty?=w390:bool)
            n134 = Index Array(array=w386) -> (element=w385:string)  [unwired: 1 in]
            n135 = Select(t=w385, s=w390, f=w389) -> (s? t:f=w384:string)
            n136 = property on="3D printer" class="CmbBox"(error in=w388, "Strings[]"=w386, "Val(Sgnl)"=w384) -> (error out=w387:errorcluster)  [unwired: 1 in, 1 out]
            n137 = case shown="False" w402 {
              tunnel: w401 -> [w413 w421]
              tunnel: [w410 w416] -> w400
              tunnel: [w406 w417] -> w399
              tunnel: w387 -> [w408 w419]
              tunnel: [w407 w421] -> w398
              tunnel: [w404 _] -> w397
              tunnel: w394 -> [_ w416]
              tunnel: w384 -> [w403 _]
              frame False {
                n138 = call-poly <vilib>:"Read Key.vi"("section"=w403, "error in (no error)"=w408, "key"="COM port", "refnum"=w413) -> ("error out"=w409:errorcluster, "value"=w411:string, "refnum out"=w407:T8)  [unwired: 4 in, 1 out]
                n139 = call <instrlib>:"Initialize.vi"("error in (no error)"=w409, "VISA resource name"=w411) -> ("error out"=w406:errorcluster, "VISA resource name out"=w410:refnum<visa-resource-name>)  [unwired: 8 in]
                n140 = Unbundle By Name(w406) -> ("status"=w405:bool)
                n141 = Not(x=w405) -> (.not. x?=w404:bool)
              }
              frame True {
                n142 = flat-sequence {
                  tunnel: [w427] -> w420
                  tunnel: w419 -> [w427]
                  frame #0 {
                    n143 = One Button Dialog(message="No printers are configured yet") -> ()  [unwired: 1 in, 1 out]
                  }
                }
                n144 = property on="Tab Control" class="TabCtl (strict)"(error in=w420) -> (error out=w418:errorcluster, "Pages"=w415:refnum<vi>[])  [unwired: 1 in, 1 out]
                n145 = for {
                  tunnel: w415 -> [w426] mode=indexing
                  tunnel: [w422] -> w414
                  i -> [w422]
                  stop <- w423 stop-if-true
                  n146 = property class="Page"(reference=w426) -> ("PageLabel"=w425:string)  [unwired: 1 in, 2 out]
                  n147 = Equal?(x=w425, y="Settings") -> (x = y?=w423:bool)
                }
                n148 = property on="Tab Control" class="TabCtl (strict)"(error in=w418, "Val(Sgnl)"=w414) -> (error out=w417:errorcluster)  [unwired: 1 in, 1 out]
              }
            }
          }
          frame "update_printer" {
            w434 = 0.0 ("X Scale.Range:Minimum")
            # "This updates the data stored in the configuration file of the selected printer. The build size is used to determine the maximum scale of the XY graph."
            n149 = Unbundle By Name(w458) -> ("data"=w460:variant)
            n150 = Variant To Data(error in=w457, type="", Variant=w460) -> (data=w448:string, error out=w456:errorcluster)
            n151 = call-poly <vilib>:"Read Key.vi"("section"=w448, "error in (no error)"=w456, "key"="COM port", "refnum"=w455) -> ("error out"=w449:errorcluster, "value"=w441:string, "refnum out"=w450:T8)  [unwired: 4 in, 1 out]
            n152 = property on="COM port" class="VISAName"("Val(Sgnl)"=w441) -> ()  [unwired: 2 in, 2 out]
            n153 = for {
              tunnel: string[] ["X_max", "Y_max", "Z_max"] -> [w467] mode=indexing
              shift-right: [w464] -> w443
              shift-left: w449 -> [w465]
              shift-right: [w463] -> w445
              shift-left: w450 -> [w466]
              tunnel: [w462] -> w453 mode=indexing
              tunnel: w448 -> [w461]
              n154 = call-poly <vilib>:"Read Key.vi"("section"=w461, "error in (no error)"=w465, "key"=w467, "refnum"=w466) -> ("error out"=w464:errorcluster, "value"=w462:dbl, "refnum out"=w463:T8)  [unwired: 4 in, 1 out]
            }
            n155 = Equal?(x=w441, y=w440) -> (x = y?=w438:bool)
            n156 = And(x=w439, y=w438) -> (x .and. y?=→"Initialized":bool)
            n157 = call <vilib>:"Get Section Names.vi"("error in (no error)"=w443, "refnum"=w445) -> ("error out"=w447:errorcluster, "section names"=w446:string[], "refnum out"=w444:T8)  [unwired: 7 in]
            n158 = Index Array(array=w453) -> (element #1=w433:dbl, element #2=w432:dbl, element #3=w452:dbl)  [unwired: 3 in]
            n159 = property on="X" class="DigNum (strict)"("Val(Sgnl)"=w433) -> ()  [unwired: 2 in, 2 out]
            n160 = property on="Y" class="DigNum (strict)"("Val(Sgnl)"=w432) -> ()  [unwired: 2 in, 2 out]
            n161 = property on="Z" class="DigNum (strict)"("Val(Sgnl)"=w452) -> ()  [unwired: 2 in, 2 out]
            n162 = property on="3D printer" class="CmbBox"(error in=w447, "Strings[]"=w446) -> (error out=w442:errorcluster)  [unwired: 1 in, 1 out]
            n163 = property on="XY Graph" class="XYGraph (strict)"("XScale.Minimum"=w434, "YScale.Minimum"=w434, "XScale.Maximum"=w433, "YScale.Maximum"=w432) -> ()  [unwired: 2 in, 2 out]
          }
          frame "save" {
            # "If a new printer is added or a value has changed it can be stored in the configuration file."
            n164 = Unbundle By Name(w482) -> ("data"=w481:variant)
            n165 = Variant To Data(error in=w479, type="", Variant=w481) -> (data=w477:string, error out=w478:errorcluster)
            n166 = call-poly <vilib>:"Write Key.vi"("section"=w477, "error in (no error)"=w478, "value"="COM port", "key"="COM port", "refnum"=w496) -> ("error out"=w487:errorcluster, "refnum out"=w488:T8)  [unwired: 4 in, 1 out]
            n167 = Build Array("X", "Y", "Z") -> (w490:dbl[])
            n168 = for {
              tunnel: w490 -> [w513] mode=indexing
              tunnel: string[] ["X_max", "Y_max", "Z_max"] -> [w512] mode=indexing
              shift-right: [w509] -> w484
              shift-left: w487 -> [w510]
              shift-right: [w508] -> w486
              shift-left: w488 -> [w511]
              tunnel: w477 -> [w507]
              n169 = call-poly <vilib>:"Write Key.vi"("section"=w507, "error in (no error)"=w510, "value"=w513, "key"=w512, "refnum"=w511) -> ("error out"=w509:errorcluster, "refnum out"=w508:T8)  [unwired: 4 in, 1 out]
            }
            n170 = Two Button Dialog(message="Reinitialize port?", 1:"No" ("F button name (\"Cancel\")"), 2:"Yes" ("T button name (\"OK\")")) -> (T button?=w473:bool)
            n171 = case shown="True" w473 {
              tunnel: w485 -> [_ w506]
              tunnel: w484 -> [w499 w505]
              tunnel: [w499 w504] -> w483
              tunnel: w477 -> [_ w500]
              frame False {
              }
              frame True {
                n172 = Bundle(cluster=T4 {"message"="", "data"=variant}, "message"="initialize", "data"=w500) -> (w501:T4)
                n173 = Enqueue Element(queue=w506, element=w501, error in (no error)=w505) -> (error out=w504:errorcluster)  [unwired: 1 in, 2 out]
              }
            }
          }
          frame "delete" {
            # "The selected printer is deleted from the configuration file."
            n174 = Unbundle By Name(w525) -> ("data"=w530:variant)
            n175 = Variant To Data(error in=w528, type="", Variant=w530) -> (data=w526:string, error out=w527:errorcluster)
            n176 = call <vilib>:"Remove Section.vi"("section"=w526, "error in (no error)"=w527, "refnum"=w531) -> ("error out"=w521:errorcluster, "refnum out"=w522:T8)  [unwired: 6 in, 1 out]
            n177 = call <vilib>:"Get Section Names.vi"("error in (no error)"=w521, "refnum"=w522) -> ("error out"=w524:errorcluster, "section names"=w523:string[], "refnum out"=w520:T8)  [unwired: 7 in]
            n178 = property on="3D printer" class="CmbBox"(error in=w524, "Strings[]"=w523) -> (error out=w519:errorcluster)  [unwired: 1 in, 1 out]
          }
          frame "move" {
            # "This is for moving the printer manually and it works easiest in relative mode. Otherwise the current position must be requested or stored."
            n179 = Unbundle By Name(w552) -> ("data"=w551:variant)
            n180 = Variant To Data(error in=w547, type=T10 {"E"=0.0, "F"=0.0, "X"=0.0, "Y"=0.0, "Z"=0.0} ("Distances"), Variant=w551) -> (data=w549:T10, error out=w543:errorcluster)
            n181 = call <instrlib>:"Positioning.vi"("error in (no error)"=w543, "type"=enum16{"Absolute (G90)", "Relative (G91)"}."Relative (G91)", "VISA resource name"=w541) -> ("error out"=w542:errorcluster, "VISA resource name out"=w540:refnum<visa-resource-name>)  [unwired: 7 in]
            n182 = call <instrlib>:"Move.vi"("error in (no error)"=w542, "Distances"=w549, "VISA resource name"=w540) -> ("error out"=w548:errorcluster, "VISA resource name out"=w546:refnum<visa-resource-name>)  [unwired: 7 in]
          }
          frame "disable_steppers" {
            # "The disable steppers command is sent to the printer."
            n183 = call <instrlib>:"Disable steppers.vi"("error in (no error)"=w556, "VISA resource name"=w557) -> ("error out"=w555:errorcluster, "VISA resource name out"=w554:refnum<visa-resource-name>)  [unwired: 8 in]
          }
          frame "home" {
            # "The home command is sent to the printer together with the axes to be homed."
            n184 = Unbundle By Name(w574) -> ("data"=w576:variant)
            n185 = Variant To Data(error in=w575, type=T11 {"X"=FALSE, "Y"=FALSE, "Z"=FALSE} ("Axes"), Variant=w576) -> (data=w572:T11, error out=w571:errorcluster)
            n186 = call <instrlib>:"Home.vi"("error in (no error)"=w571, "Axes"=w572, "VISA resource name"=w577) -> ("error out"=w569:errorcluster, "VISA resource name out"=w570:refnum<visa-resource-name>)  [unwired: 7 in]
          }
          frame "set_temp" {
            # "The temperature of the selected heater is set to the set temperature."
            n187 = Unbundle By Name(w591) -> ("data"=w590:variant)
            n188 = Variant To Data(error in=w582, type=cluster{"setpoint":i32, "Heater":T9} {"setpoint"=0, "Heater"=enum."Hot end"} ("output cluster"), Variant=w590) -> (data=w588:cluster{"setpoint":i32, "Heater":T9}, error out=w581:errorcluster)
            n189 = Unbundle(w588) -> ("setpoint"=w587:i32, "Heater"=w586:T9)
            n190 = call <instrlib>:"Set temperature.vi"("error in (no error)"=w581, "Heater"=w586, "Temperature"=w587, "VISA resource name"=w585) -> ("error out"=w583:errorcluster, "VISA resource name out"=w584:refnum<visa-resource-name>)  [unwired: 6 in]
          }
          frame "set_fan" {
            # "Sets the fan speed."
            n191 = Unbundle By Name(w607) -> ("data"=w606:variant)
            n192 = Variant To Data(error in=w602, type=u8 0 ("Fan speed"), Variant=w606) -> (data=w599:u8, error out=w601:errorcluster)
            n193 = call <instrlib>:"Set fan speed.vi"("error in (no error)"=w601, "Fan speed"=w599, "VISA resource name"=w605) -> ("error out"=w603:errorcluster, "VISA resource name out"=w604:refnum<visa-resource-name>)  [unwired: 7 in]
          }
          frame "request_data" {
            # "This case is triggered by the timed loop. Another option would be to send a message to itself, but that causes a delay."
            n194 = call <instrlib>:"Get Endstop Status.vi"("error in (no error)"=w616, "VISA resource name"=w631) -> ("error out"=w619:errorcluster, "End stop status"=w625:T12, "VISA resource name out"=w621:refnum<visa-resource-name>)  [unwired: 7 in]
            n195 = Unbundle(w625) -> ("x_min"=→"X min":bool, "y_min"=→"Y min":bool, "z_min"=→"Z min":bool)
            n196 = call <instrlib>:"Report temperatures.vi"("error in (no error)"=w619, "VISA resource name"=w621) -> ("error out"=w614:errorcluster, "Temperatures"=w620:T13, "VISA resource name out"=w630:refnum<visa-resource-name>)  [unwired: 7 in]
            n197 = Cluster To Array(cluster=w620) -> (array=w618:dbl[])
            n198 = Build Array(w618) -> (→"Temperature Chart":dbl[][])
          }
          frame "load_gcode" {
            # "The gcode file is loaded wron the selected path and is converted to an array of strings. This array is used to iterate through all gcodes."
            n199 = Unbundle By Name(w649) -> ("data"=w648:variant)
            n200 = Variant To Data(error in=w644, type=path "", Variant=w648) -> (data=w646:path, error out=w645:errorcluster)
            n201 = call "read Gcode.vi"("error in"=w645, "Gcode path (use dialog)"=w646) -> ("error out"=w636:errorcluster, "Gcode Array"=w637:string[])  [unwired: 7 in, 1 out]
            "Gcode array" <- w637
            n202 = property on="Gcode array" class="Arr (strict)"(error in=w636, "Index Values"=u32[] []) -> (error out=w635:errorcluster)  [unwired: 1 in, 1 out]
            n203 = property on="Start Gcode" class="Bool"(error in=w635, "DisabledEnum"=T3."Enabled" ("Disabled")) -> (error out=w639:errorcluster)  [unwired: 1 in, 1 out]
          }
          frame "run_gcode" {
            # "This case runs the indexed gcode from the gcode array. The index is increased by one every time this case is selected. The data is filetered and put in an XY graph because that's just awesome."
            n204 = Unbundle By Name(w684) -> ("data"=w685:variant)
            n205 = Array Size(array=w674) -> (size(s)=w672:i32)
            n206 = Variant To Data(error in=w683, type=0, Variant=w685) -> (data=w663:i32, error out=w680:errorcluster)
            n207 = Greater Or Equal?(x=w663, y=w672) -> (x >= y?=w671:bool)
            n208 = Increment(x=w663) -> (x+1=w662:i32)
            n209 = Index Array(array=w674, index=w663) -> (element=w666:string)
            n210 = call "build XY graph.vi"("Gcode line"=w666, "XY Graph in"=w667) -> ("XY Graph out"=w665:cluster{"X":dbl, "Y":dbl}[])  [unwired: 5 in]
            "XY Graph" <- w665
            n211 = Subtract(x=w662, y=7) -> (x-y=w659:i32)
            n212 = case shown="True" "Test mode" {
              tunnel: w681 -> [w692 w695]
              tunnel: w680 -> [w691 w694]
              tunnel: [w690 w695] -> w679
              tunnel: [w689 w694] -> _
              tunnel: w666 -> [w688 _]
              frame False {
                n213 = call <instrlib>:"Send raw Gcode.vi"("error in (no error)"=w691, "Gcode"=w688, "VISA resource name"=w692) -> ("error out"=w689:errorcluster, "VISA resource name out"=w690:refnum<visa-resource-name>)  [unwired: 5 in, 2 out]
              }
              frame True {
                n214 = Wait (ms)(milliseconds to wait=u32 0) -> ()  [unwired: 1 out]
              }
            }
            n215 = Less Or Equal To 0?(x=w659) -> (x <= 0?=w660:bool)
            n216 = Select(t=0, s=w660, f=w659) -> (s? t:f=w654:i32)
            n217 = Build Array(w654) -> (w653:i32[])
            n218 = property on="Gcode array" class="Arr (strict)"("Index Values"=w653) -> ()  [unwired: 2 in, 2 out]
            n219 = Increment(x=w663) -> (x+1=w673:i32)
            n220 = Select(t="finish_gcode" ("message"), s=w671, f="run_gcode" ("message")) -> (s? t:f=w668:string)
            n221 = Bundle(cluster=T4 {"message"="", "data"=variant} ("element"), "message"=w668, "data"=w673) -> (w677:T4)
            n222 = Enqueue Element(queue=w675, element=w677) -> (error out=w676:errorcluster)  [unwired: 2 in, 2 out]
          }
          frame "pause_gcode" {
            # "The pause gcode flushes the queue to prevent further messages from performing. The Z is raised by 5mm and the hotend can be moved with the manual controls if needed. If the pause button is selected again all flushed queue elements are put back into the queue and the gcode will run where it left off."
            n223 = Not(x=w705) -> (.not. x?=w703:bool)
            n224 = case shown="True" w703 {
              tunnel: w704 -> [w714 w725]
              tunnel: [w711 w724] -> w702
              tunnel: w701 -> [w711 _]
              tunnel: w700 -> [w713 w722]
              tunnel: [w712 w723] -> w699
              tunnel: w697 -> [w710 w721]
              tunnel: [w710 w720] -> w696
              frame False {
                n225 = for {
                  tunnel: w714 -> [w718]
                  tunnel: w711 -> [w717] mode=indexing
                  shift-right: [w715] -> w712
                  shift-left: w713 -> [w716]
                  n226 = Enqueue Element(queue=w718, element=w717, error in (no error)=w716) -> (error out=w715:errorcluster)  [unwired: 1 in, 2 out]
                }
              }
              frame True {
                n227 = property on="Test mode" class="Bool (strict)"() -> ("Value"=w719:bool)  [unwired: 2 in, 2 out]
                n228 = Flush Queue(queue=w725, error in (no error)=w722) -> (remaining elements=w724:T4[], error out=w723:errorcluster)  [unwired: 1 out]
                n229 = case shown="False" w719 {
                  tunnel: w721 -> [w735 w737]
                  tunnel: [w727 w737] -> w720
                  frame False {
                    n230 = call <instrlib>:"Positioning.vi"("type"=enum16{"Absolute (G90)", "Relative (G91)"}."Relative (G91)", "VISA resource name"=w735) -> ("error out"=w733:errorcluster, "VISA resource name out"=w736:refnum<visa-resource-name>)  [unwired: 8 in]
                    n231 = Bundle By Name(cluster=T10 {"E"=0.0, "F"=0.0, "X"=0.0, "Y"=0.0, "Z"=0.0} ("Distances"), "Z"=5.0) -> (w728:T10)
                    n232 = call <instrlib>:"Move.vi"("error in (no error)"=w733, "Distances"=w728, "VISA resource name"=w736) -> ("error out"=w732:errorcluster, "VISA resource name out"=w731:refnum<visa-resource-name>)  [unwired: 7 in]
                    n233 = call <instrlib>:"Positioning.vi"("error in (no error)"=w732, "type"=enum16{"Absolute (G90)", "Relative (G91)"}."Absolute (G90)", "VISA resource name"=w731) -> ("VISA resource name out"=w727:refnum<visa-resource-name>)  [unwired: 7 in, 1 out]
                  }
                  frame True {
                  }
                }
              }
            }
          }
          frame "stop_gcode" {
            (unwired) 0 ("Top Row")
            (unwired) string[] [] ("Item Names")
            w740 = T3."Disabled and Grayed Out" ("Disabled")
            # "The gcode is stopped and the queue is flushed and forgotten to prevent further actions."
            n234 = Flush Queue(queue=w744, error in (no error)=w743) -> (error out=w742:errorcluster)  [unwired: 2 out]
            n235 = invoke on="Gcode file" class="Path" method="Reinit To Default"() -> ()  [unwired: 3 in, 3 out]
            n236 = invoke on="XY Graph" class="XYGraph (strict)" method="Reinit To Default"() -> ()  [unwired: 3 in, 3 out]
            n237 = property on="Gcode array" class="Arr (strict)"("Index Values"=u32[] []) -> ()  [unwired: 2 in, 2 out]
            n238 = property on="Pause Gcode" class="Bool"("DisabledEnum"=w740) -> ()  [unwired: 2 in, 2 out]
            n239 = property on="Stop Gcode" class="Bool"("DisabledEnum"=w740) -> ()  [unwired: 2 in, 2 out]
            n240 = property on="Start Gcode" class="Bool"("DisabledEnum"=w740) -> ()  [unwired: 2 in, 2 out]
          }
          frame "finish_gcode" {
            (unwired) 0 ("Top Row")
            (unwired) string[] [] ("Item Names")
            w751 = T3."Disabled and Grayed Out" ("Disabled")
            # "The gcode is stopped but on a positive note."
            n241 = invoke on="Gcode file" class="Path" method="Reinit To Default"() -> ()  [unwired: 3 in, 3 out]
            n242 = invoke on="XY Graph" class="XYGraph (strict)" method="Reinit To Default"() -> ()  [unwired: 3 in, 3 out]
            n243 = property on="Gcode array" class="Arr (strict)"("Index Values"=u32[] []) -> ()  [unwired: 2 in, 2 out]
            n244 = One Button Dialog(message="Gcode finished!") -> ()  [unwired: 1 in, 1 out]
            n245 = property on="Pause Gcode" class="Bool"("DisabledEnum"=w751) -> ()  [unwired: 2 in, 2 out]
            n246 = property on="Stop Gcode" class="Bool"("DisabledEnum"=w751) -> ()  [unwired: 2 in, 2 out]
            n247 = property on="Start Gcode" class="Bool"("DisabledEnum"=w751) -> ()  [unwired: 2 in, 2 out]
          }
          frame "start_torture" {
            # "The torture sequence is started. The printer is homed after which the head is placed into the center at a Z height of 10mm. The torture sequence is selected."
            n248 = case shown="False" "Test mode" {
              tunnel: w770 -> [w788 w809]
              tunnel: w769 -> [w787 w810]
              tunnel: "Axle" -> [w784 _]
              tunnel: [w778 w810] -> w763
              tunnel: [w777 w809] -> w762
              frame False {
                n249 = property on="Distance" class="Slide (strict)"() -> ("Value"=w785:dbl)  [unwired: 2 in, 2 out]
                n250 = property on="X" class="DigNum (strict)"() -> ("Value"=w797:dbl)  [unwired: 2 in, 2 out]
                n251 = property on="Y" class="DigNum (strict)"() -> ("Value"=w794:dbl)  [unwired: 2 in, 2 out]
                n252 = Divide(x=w797, y=2.0) -> (x/y=w782:dbl)
                n253 = Divide(x=w794, y=2.0) -> (x/y=w780:dbl)
                n254 = Divide(x=w785, y=2.0) -> (x/y=w779:dbl)
                n255 = case shown="\"Y\"" w784 {
                  tunnel: [w802 w808] -> w783
                  tunnel: w782 -> [w803 w808]
                  tunnel: w779 -> [w804 _]
                  tunnel: [w801 w805] -> w781
                  tunnel: w780 -> [w801 w806]
                  tunnel: w779 -> [_ w807]
                  frame "X", Default {
                    n256 = Subtract(x=w803, y=w804) -> (x-y=w802:dbl)
                  }
                  frame "Y" {
                    n257 = Subtract(x=w806, y=w807) -> (x-y=w805:dbl)
                  }
                }
                n258 = call <instrlib>:"Home.vi"("error in (no error)"=w787, "VISA resource name"=w788) -> ("error out"=w790:errorcluster, "VISA resource name out"=w789:refnum<visa-resource-name>)  [unwired: 8 in]
                n259 = call <instrlib>:"Positioning.vi"("error in (no error)"=w790, "type"=enum16{"Absolute (G90)", "Relative (G91)"}."Absolute (G90)", "VISA resource name"=w789) -> ("error out"=w799:errorcluster, "VISA resource name out"=w800:refnum<visa-resource-name>)  [unwired: 7 in]
                n260 = Bundle By Name(cluster=T10 {"E"=0.0, "F"=0.0, "X"=0.0, "Y"=0.0, "Z"=0.0} ("Distances"), "X"=w783, "Y"=w781, "Z"=10.0) -> (w791:T10)
                n261 = call <instrlib>:"Move.vi"("error in (no error)"=w799, "Distances"=w791, "VISA resource name"=w800) -> ("error out"=w778:errorcluster, "VISA resource name out"=w777:refnum<visa-resource-name>)  [unwired: 7 in]
              }
              frame True {
              }
            }
            n262 = Enqueue Element(queue=w766, element=T4 {"message"="torture", "data"=variant}, error in (no error)=w763) -> (error out=w764:errorcluster)  [unwired: 1 in, 2 out]
          }
          frame "torture" {
            # "This sequence moves the print head symmetric from the bed center back and forth without waiting. The frequence can be changed by changing the travel distance or movement speed. This case calls itself to stay in a loop."
            n263 = Divide(x="Distance", y=2.0) -> (x/y=w817:dbl)
            n264 = property on="Axle" class="Enum (strict)"() -> ("Value"=w820:enum16{"X", "Y", "Z"})  [unwired: 2 in, 2 out]
            n265 = case shown="\"Y\"" w820 {
              tunnel: T10 {"E"=0.0, "F"=0.0, "X"=0.0, "Y"=0.0, "Z"=0.0} ("Distances") -> [w855 w865]
              tunnel: [w854 w866] -> w829
              tunnel: "Speed" -> [w853 w864]
              tunnel: w817 -> [w847 w858]
              tunnel: w816 -> [w849 w860]
              tunnel: [w846 w857] -> w812
              tunnel: [w845 w856] -> w811
              frame "X", Default {
                n266 = property on="X" class="DigNum (strict)"() -> ("Value"=w846:dbl)  [unwired: 2 in, 2 out]
                n267 = Divide(x=w846, y=2.0) -> (x/y=w848:dbl)
                n268 = Add(x=w848, y=w847) -> (x+y=w851:dbl)
                n269 = Subtract(x=w848, y=w847) -> (x-y=w850:dbl)
                n270 = Select(t=w851, s=w849, f=w850) -> (s? t:f=w845:dbl)
                n271 = Bundle By Name(cluster=w855, "F"=w853, "X"=w845) -> (w854:T10)
              }
              frame "Y" {
                n272 = property on="Y" class="DigNum (strict)"() -> ("Value"=w857:dbl)  [unwired: 2 in, 2 out]
                n273 = Divide(x=w857, y=2.0) -> (x/y=w859:dbl)
                n274 = Add(x=w859, y=w858) -> (x+y=w862:dbl)
                n275 = Subtract(x=w859, y=w858) -> (x-y=w861:dbl)
                n276 = Select(t=w862, s=w860, f=w861) -> (s? t:f=w856:dbl)
                n277 = Bundle By Name(cluster=w865, "F"=w864, "Y"=w856) -> (w866:T10)
              }
            }
            "Position sent" <- w811
            n278 = Not(x=w816) -> (.not. x?=w815:bool)
            n279 = property on="Test mode" class="Bool (strict)"() -> ("Value"=w814:bool)  [unwired: 2 in, 2 out]
            n280 = case shown="False" w814 {
              tunnel: w829 -> [w841 _]
              tunnel: w828 -> [w840 w843]
              tunnel: w827 -> [w839 w842]
              tunnel: [w838 w842] -> w826
              tunnel: [w837 w843] -> w824
              frame False {
                n281 = call <instrlib>:"Move.vi"("error in (no error)"=w840, "Distances"=w841, "VISA resource name"=w839) -> ("error out"=w837:errorcluster, "VISA resource name out"=w838:refnum<visa-resource-name>)  [unwired: 7 in]
              }
              frame True {
                n282 = Wait (ms)(milliseconds to wait=u32 10) -> ()  [unwired: 1 out]
              }
            }
            n283 = property on="Distance" class="Slide (strict)"("Scale.Minimum"=0.0 ("Scale.Range:Minimum"), "Scale.Maximum"=w812) -> ()  [unwired: 2 in, 2 out]
            n284 = Enqueue Element(queue=w822, element=T4 {"message"="torture", "data"=variant}, error in (no error)=w824) -> (error out=w823:errorcluster)  [unwired: 1 in, 2 out]
          }
          frame "stop_torture" {
            # "The queue is flushed so the remaining torture messages aren't performed anymore."
            n285 = Flush Queue(queue=w869, error in (no error)=w868) -> (error out=w867:errorcluster)  [unwired: 2 out]
          }
          frame "close" {
            # "This closes the port and ends the loop."
            n286 = call <instrlib>:"Close.vi"("error in (no error)"=w879, "VISA resource name"=w880) -> ("error out"=w878:errorcluster)  [unwired: 9 in]
          }
        }
      }
      frame Error {
        # "This case is selected when the Dequeue element generates an error. This means that the queue is released and the close message is sent to select the close case."
        n287 = Enqueue Element(queue=w890, element=T4 {"message"="close", "data"=variant}) -> (error out=w889:errorcluster)  [unwired: 2 in, 2 out]
      }
    }
    n288 = call <vilib>:"Clear Errors.vi"("error in (no error)"=w330, "specific error code to clear (0: all)"=1) -> ("error out"=w329:errorcluster)  [unwired: 4 in, 1 out]
    n289 = call <vilib>:"Simple Error Handler.vi"("error in (no error)"=w329) -> ("error out"=w323:errorcluster)  [unwired: 4 in, 4 out]
  }
  n290 = node-c288(w21) -> ()  [unwired: 1 out]
  n291 = Release Queue(queue=w38, error in (no error)=w39) -> ()  [unwired: 1 in, 3 out]
  n292 = call <vilib>:"Close Config Data.vi"("error in (no error)"=w27, "refnum"=w29) -> ("error out"=w10:errorcluster)  [unwired: 8 in, 1 out]
  n293 = property class="VI"(error in=w10, "Front Panel Window:Open"=FALSE) -> ()  [unwired: 1 in, 2 out]
